vi "Generate Simulated Data.vi"(8 "error in (no error)":T2 caption="entrée d'erreur (pas d'erreur)", 11 "Type de signal":T1) -> (0 "error out":T2 caption="sortie d'erreur", 2 "Données du graphe":waveform(dbl)[](array[waveform]))   [LabVIEW 2020, in "Acquisition.lvlib"]
doc: "Génère des exemples de waveforms en fonction du type de signal dans l'entrée Configuration du matériel."
uses:
  Acquisition.lvlib
  Signal Type.ctl
  <vilib>/Analysis/NI_AALBase.lvlib
panel:
  out "Tableau des médianes 2":dbl[](array[numeric])
  out "Tableau des médianes":dbl[](array[numeric])
  in  "S5":bool[](array[boolean])=[FALSE, TRUE, FALSE, TRUE]
  in  "S4":bool[](array[boolean])=[FALSE, TRUE, FALSE, FALSE]
  in  "S6":bool[](array[boolean])=[FALSE, TRUE, TRUE, FALSE]
  in  "S7":bool[](array[boolean])=[FALSE, TRUE, TRUE, TRUE]
  in  "S13":bool[](array[boolean])=[TRUE, TRUE, FALSE, TRUE]
  in  "S12":bool[](array[boolean])=[TRUE, TRUE, FALSE, FALSE]
  in  "S11":bool[](array[boolean])=[TRUE, FALSE, TRUE, TRUE]
  in  "S10":bool[](array[boolean])=[TRUE, FALSE, TRUE, FALSE]
  in  "S9":bool[](array[boolean])=[TRUE, FALSE, FALSE, TRUE]
  in  "S8":bool[](array[boolean])=[TRUE, FALSE, FALSE, FALSE]
  in  "stop":bool
  in  "S3":bool[](array[boolean])=[TRUE, TRUE, FALSE, FALSE]
  in  "S2":bool[](array[boolean])=[FALSE, TRUE, FALSE, FALSE]
  in  "S1":bool[](array[boolean])=[TRUE, FALSE, FALSE, FALSE]
  in  "S0":bool[](array[boolean])=[FALSE, FALSE, FALSE, FALSE]
  in  "nom du périphérique":tag="Dev1"
  out "Graphe déroulant":dynamicdata(graph)
  out "Affiche la médiane":dbl
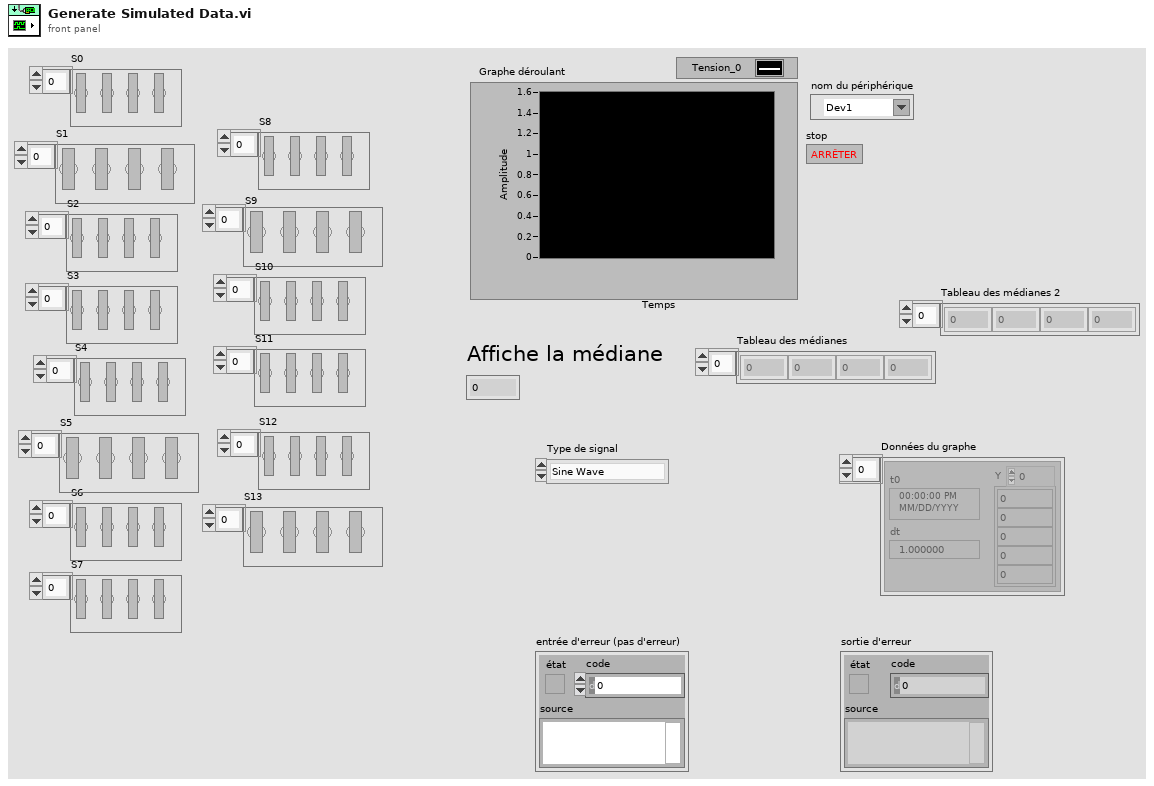
[diagram p1: front panel]
types:
  T1 = typedef "Acquisition.lvlib/Signal Type.ctl" = enum16{"Sine Wave", "Square with Noise", "Signal triangulaire", "Simulation DAQ"}
  T2 = cluster{"état":bool, "code":i32, "source":string}
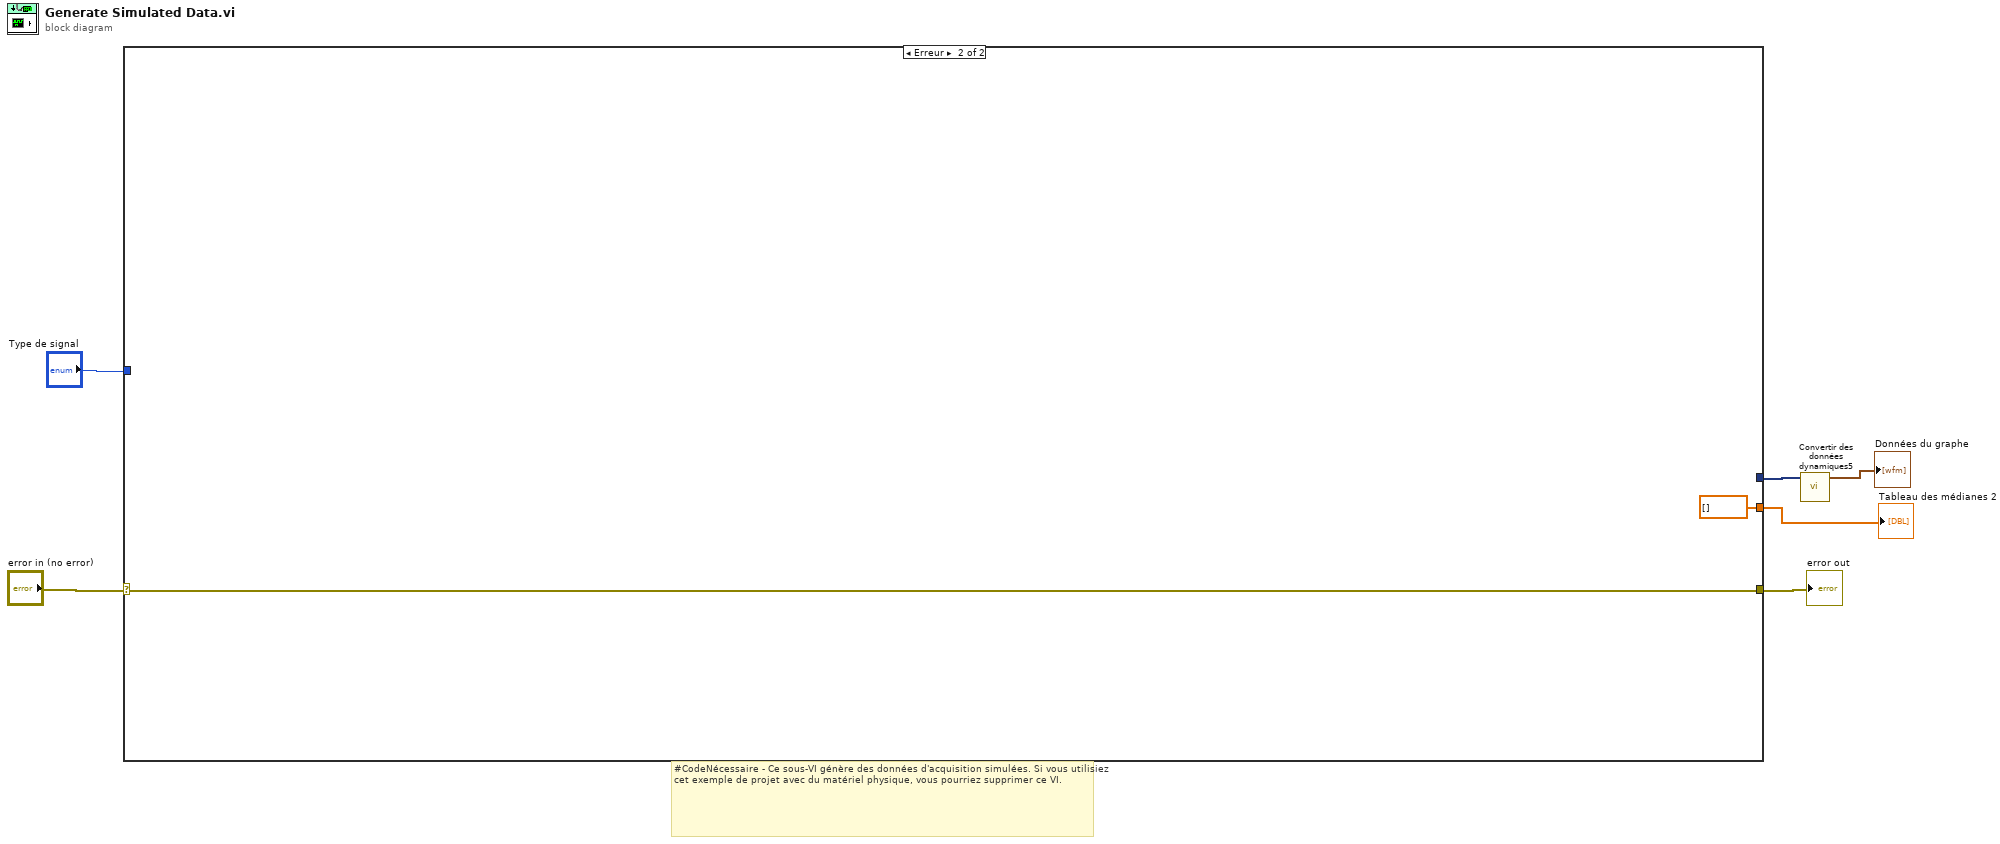
[diagram p0: block diagram]
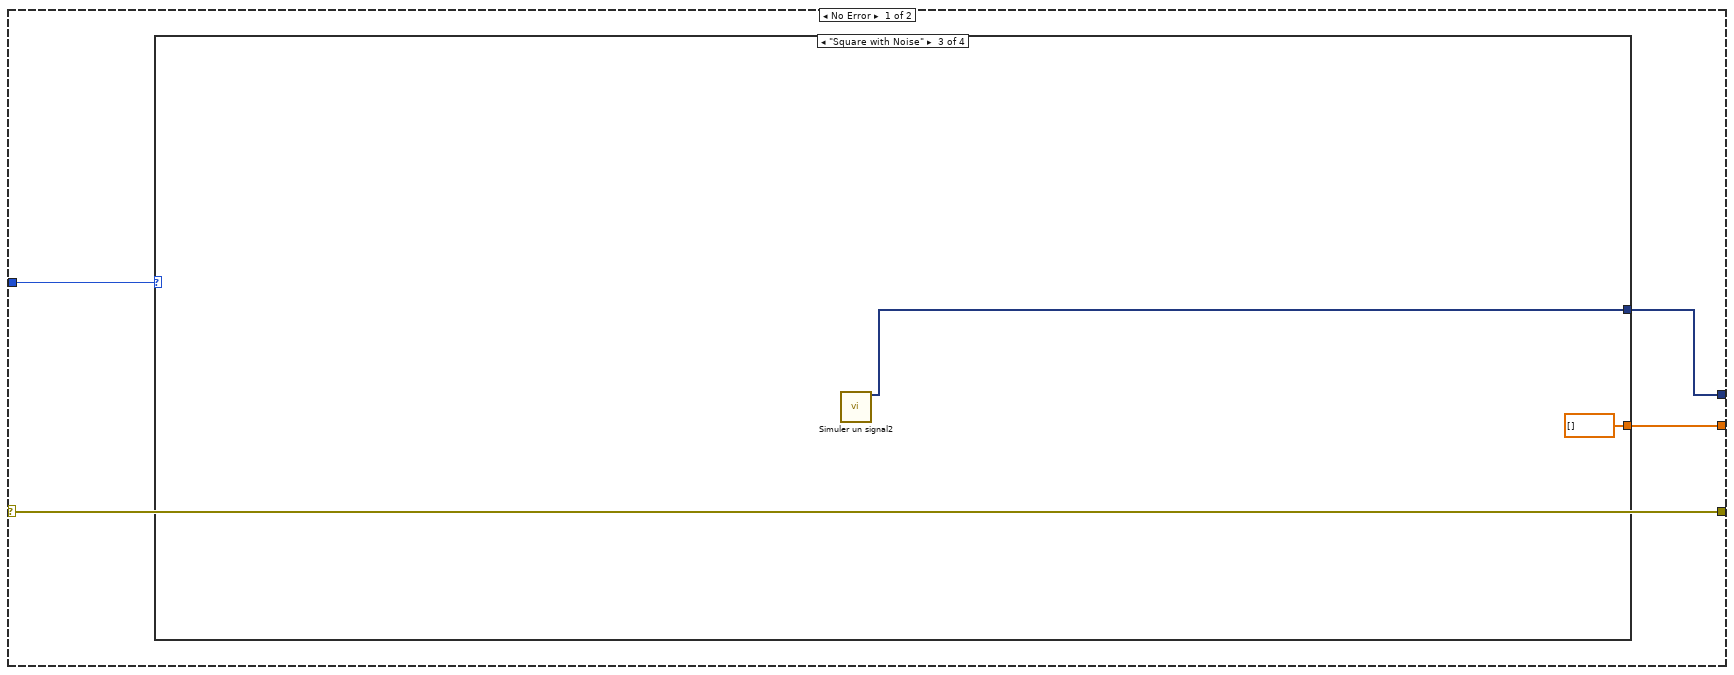
[diagram p2: hidden frame]
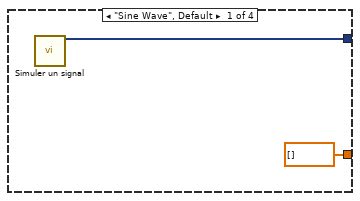
[diagram p3: hidden frame]
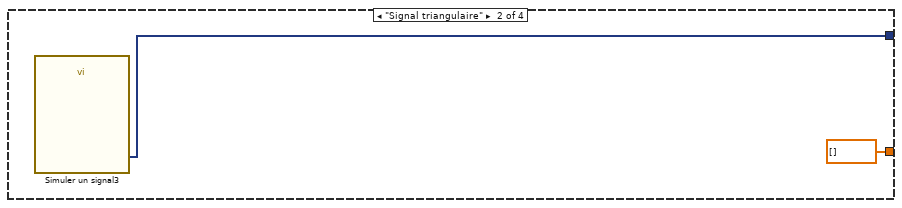
[diagram p4: hidden frame]
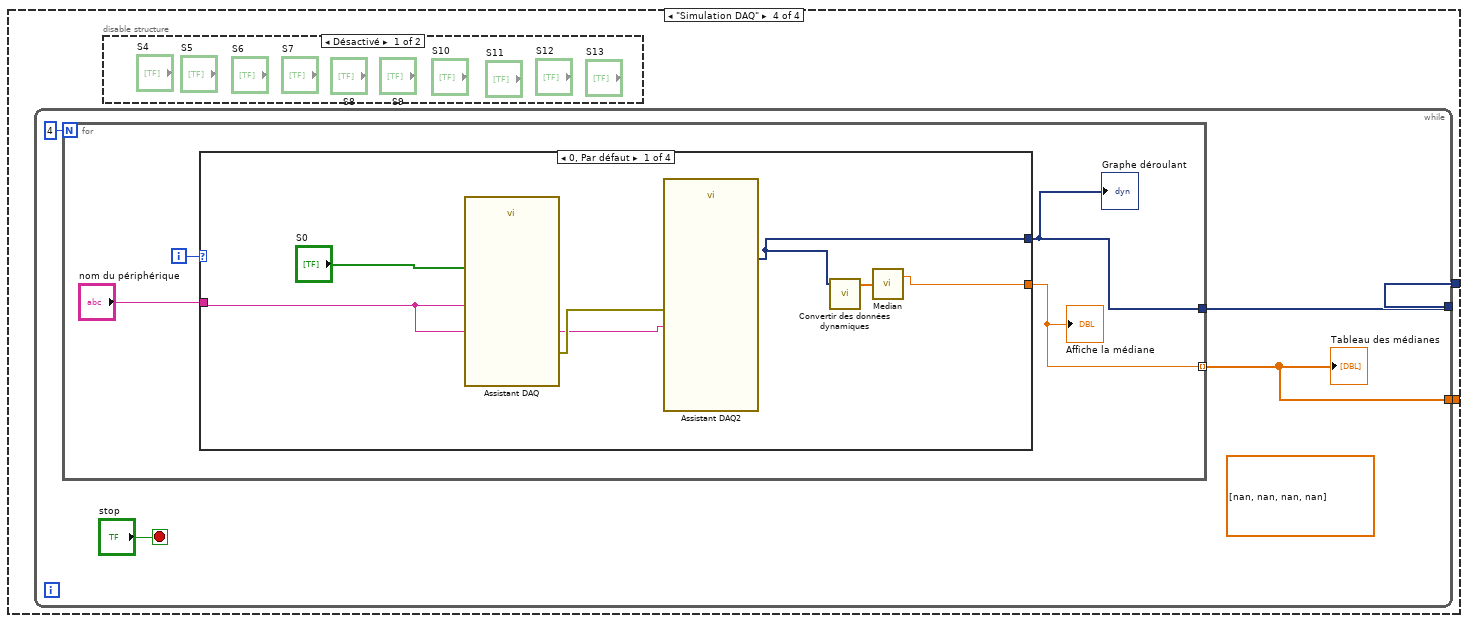
[diagram p5: hidden frame]
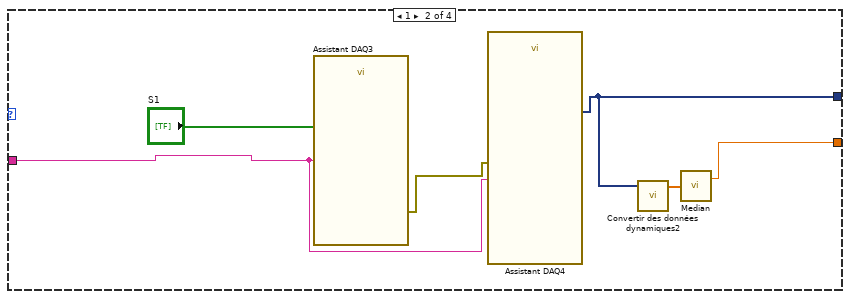
[diagram p7: hidden frame]
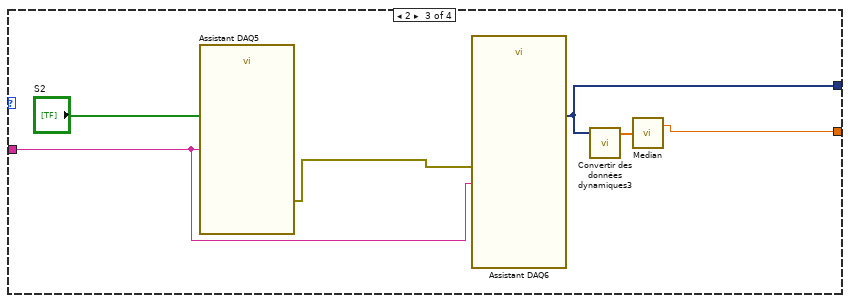
[diagram p8: hidden frame]
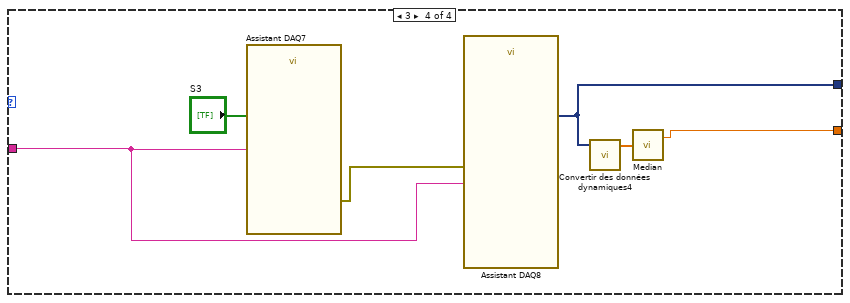
[diagram p9: hidden frame]
diagram:
  # "#CodeNécessaire - Ce sous-VI génère des données d'acquisition simulées. Si vous utilisiez cet exemple de projet avec du matériel physique, vous pourriez supprimer ce VI."
  n1 = case shown="Erreur" "error in (no error)" {
    selector: "error in (no error)" -> [w10 w52]
    tunnel: [w10 w52] -> w5
    tunnel: [w8 _] -> w4
    tunnel: "Type de signal" -> [w9 _]
    tunnel: [w7 dbl[] []] -> w1
    frame No Error {
      n2 = case shown="\"Square with Noise\"" w9 {
        tunnel: [w12 w14 w16 w18] -> w8
        tunnel: [dbl[] [] dbl[] [] dbl[] [] w17] -> w7
        frame "Sine Wave", Default {
          n3 = call "Simuler un signal"() -> ("Sine"=w12:dynamicdata)  [unwired: 14 in, 1 out]
        }
        frame "Signal triangulaire" {
          n4 = call "Simuler un signal3"() -> ("Triangle"=w14:dynamicdata)  [unwired: 14 in, 1 out]
        }
        frame "Square with Noise" {
          n5 = call "Simuler un signal2"() -> ("Square with Gaussian Noise"=w16:dynamicdata)  [unwired: 14 in, 1 out]
        }
        frame "Simulation DAQ" {
          n6 = while {
            tunnel: [w20] -> w18
            tunnel: [w19] -> w17
            stop <- "stop" stop-if-true
            (unwired) dbl[] [nan, nan, nan, nan] ("Tableau des médianes")
            n7 = for {
              N: 4 -> [_]
              tunnel: [w23] -> w19 mode=indexing
              tunnel: [w24] -> w20
              i -> [w26]
              n8 = case shown="0, Par défaut" w26 {
                tunnel: "nom du périphérique" -> [w30 w36 w42 w48]
                tunnel: [w28 w34 w40 w47] -> w24
                tunnel: [w27 w33 w39 w45] -> w23
                frame 0, Default {
                  n9 = call "Assistant DAQ"("data"="S0", "nom du périphérique"=w30) -> ("error out"=w31:errorcluster)  [unwired: 16 in, 1 out]
                  n10 = call "Assistant DAQ2"("error in"=w31, "nom du périphérique"=w30) -> ("data"=w28:dynamicdata)  [unwired: 15 in, 2 out]
                  n11 = call "Convertir des données dynamiques"("Dynamic Data Type"=w28) -> ("Array"=w29:dbl[])  [unwired: 3 in]
                  n12 = call <vilib>:"Median.vi"("X"=w29) -> ("median"=w27:dbl)  [unwired: 1 out]
                }
                frame 1 {
                  n13 = call "Assistant DAQ3"("data"="S1", "nom du périphérique"=w36) -> ("error out"=w37:errorcluster)  [unwired: 16 in, 1 out]
                  n14 = call "Assistant DAQ4"("error in"=w37, "nom du périphérique"=w36) -> ("data"=w34:dynamicdata)  [unwired: 15 in, 2 out]
                  n15 = call "Convertir des données dynamiques2"("Dynamic Data Type"=w34) -> ("Array"=w35:dbl[])  [unwired: 3 in]
                  n16 = call <vilib>:"Median.vi"("X"=w35) -> ("median"=w33:dbl)  [unwired: 1 out]
                }
                frame 2 {
                  n17 = call "Assistant DAQ5"("data"="S2", "nom du périphérique"=w42) -> ("error out"=w43:errorcluster)  [unwired: 16 in, 1 out]
                  n18 = call "Assistant DAQ6"("error in"=w43, "nom du périphérique"=w42) -> ("data"=w40:dynamicdata)  [unwired: 15 in, 2 out]
                  n19 = call "Convertir des données dynamiques3"("Dynamic Data Type"=w40) -> ("Array"=w41:dbl[])  [unwired: 3 in]
                  n20 = call <vilib>:"Median.vi"("X"=w41) -> ("median"=w39:dbl)  [unwired: 1 out]
                }
                frame 3 {
                  n21 = call "Assistant DAQ7"("data"="S3", "nom du périphérique"=w48) -> ("error out"=w49:errorcluster)  [unwired: 16 in, 1 out]
                  n22 = call "Assistant DAQ8"("error in"=w49, "nom du périphérique"=w48) -> ("data"=w47:dynamicdata)  [unwired: 15 in, 2 out]
                  n23 = call "Convertir des données dynamiques4"("Dynamic Data Type"=w47) -> ("Array"=w46:dbl[])  [unwired: 3 in]
                  n24 = call <vilib>:"Median.vi"("X"=w46) -> ("median"=w45:dbl)  [unwired: 1 out]
                }
              }
              "Affiche la médiane" <- w23
              "Graphe déroulant" <- w24
            }
            "Tableau des médianes" <- w19
          }
          n25 = disable-structure shown="Désactivé" {
            frame Disabled {
            }
            frame Enabled {
            }
          }
        }
      }
    }
    frame Error {
    }
  }
  "error out" <- w5
  "Tableau des médianes 2" <- w1
  n26 = call "Convertir des données dynamiques5"("Dynamic Data Type"=w4) -> ("Array of Waveform"=→"Données du graphe":waveform(dbl)[])  [unwired: 3 in]
